vi "Thermocouples subVI.vi"() -> (2 "data":dynamicdata(waveform), 3 "Cluster":cluster{"TC1":dbl, "TC2":dbl, "TC3":dbl})   [LabVIEW 2015]
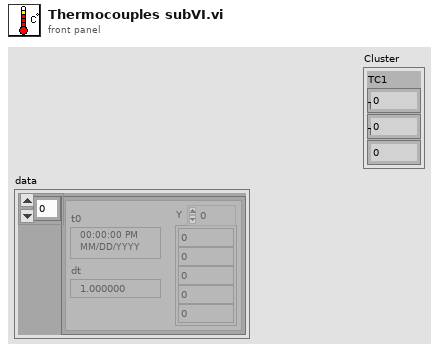
[diagram p1: front panel]
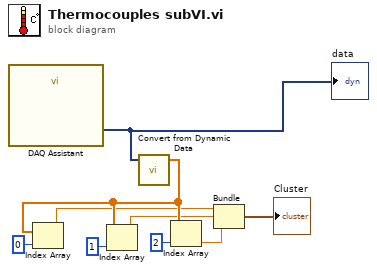
[diagram p0: block diagram]
diagram:
  n1 = call "DAQ Assistant"() -> ("data"=w9:dynamicdata)  [unwired: 17 in, 2 out]
  "data" <- w9
  n2 = call "Convert from Dynamic Data"("Dynamic Data Type"=w9) -> ("Array"=w7:dbl[])  [unwired: 3 in]
  n3 = Index Array(array=w7, index=0) -> (element=w4:dbl)
  n4 = Index Array(array=w7, index=1) -> (element=w5:dbl)
  n5 = Index Array(array=w7, index=2) -> (element=w6:dbl)
  n6 = Bundle(w4, w5, w6) -> (→"Cluster":cluster{dbl, dbl, dbl})  [unwired: 1 in]
